vi "write_image.vi"(8 "error in":errorcluster, 10 "image":u8[](array[numeric]), 11 "slmCluster":T1) -> (0 "error out":errorcluster)   [LabVIEW 2015]
uses:
  Labview/InstrumentControl20190423/slm_Meadowlark_hdmi_device.llb/slmCluster.ctl
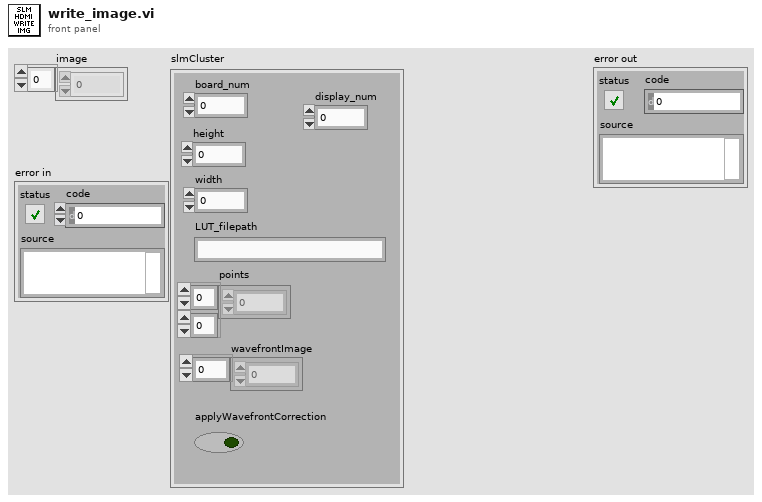
[diagram p1: front panel]
types:
  T1 = typedef "slmCluster.ctl" = cluster{"board_num":u32, "height":u32, "width":u32, "LUT_filepath":string, "points":i32[][], "wavefrontImage":u8[], "applyWavefrontCorrection":bool, "display_num":i32}
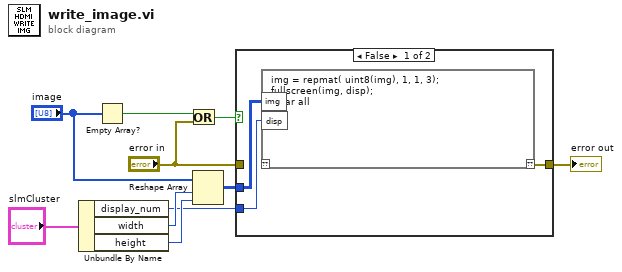
[diagram p0: block diagram]
diagram:
  n1 = Unbundle By Name("slmCluster") -> ("display_num"=w1:i32, "width"=w4:u32, "height"=w3:u32)
  n2 = Empty Array?(array="image") -> (empty?=w10:bool)
  n3 = Or(x=w10, y="error in") -> (x .or. y?=w9:bool)
  n4 = Reshape Array("image", w4, w3) -> (w2:u8[][])
  n5 = case shown="False" w9 {
    tunnel: w1 -> [w13 _]
    tunnel: [w12 w14] -> w8
    tunnel: "error in" -> [_ w14]
    tunnel: w2 -> [w11 _]
    frame False {
      n6 = script code="img = repmat( uint8(img), 1, 1, 3);\nfullscreen(img, disp);\nclear all"("img"=w11, "disp"=w13) -> ("??"=w12:errorcluster)  [unwired: 1 in]
    }
    frame True {
    }
  }
  "error out" <- w8
